vi "UIStep Execte UI Validate Input.vi"(10 "UI Setting":T1={"Embedded"=FALSE, "Size"=enum."Small", "Title"="", "Content"="", "Text Style"={"Font"="", "Size"=0.0, "Justification"=1, "TextColor"=0, "BGColor"=0, "Bold"=FALSE}, "Buttons"={"Button1"={"Label"="", "Size"=0.0, "TextColor"=0, "BGColor"=0, "Bold"=FALSE}, "Button2"={"Label"="", "Size"=0.0, "TextColor"=0, "BGColor"=0, "Bold"=FALSE}}, "Image"=path "", "Enable Input"=FALSE, "Input Validation"=""} {"Text Style"."Justification" items=["Left", "Center", "Right"]}, 11 "UI Control":T2) -> (2 "Valid out":bool, 3 "UI Control out":T2)   [LabVIEW 2015, in "UIStep.lvclass"]
uses:
  UIStep.lvclass
  <vilib>/regexp/Match Regular Expression.xnode
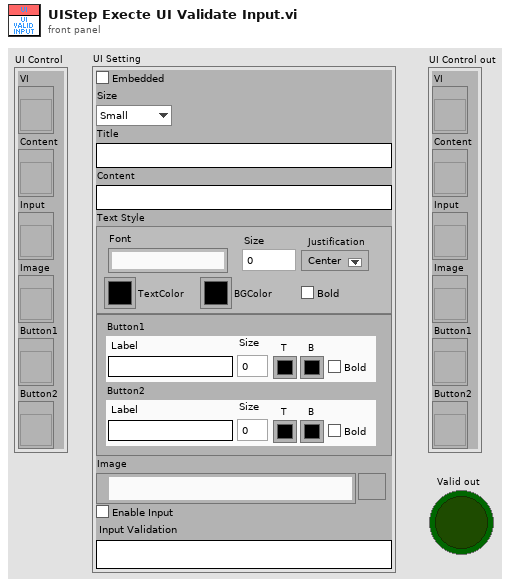
[diagram p1: front panel]
types:
  T1 = cluster{"Embedded":bool, "Size":enum16{"Small", "Middle", "Big"}, "Title":string, "Content":string, "Text Style":cluster{"Font":string, "Size":dbl, "Justification":u16, "TextColor":u32, "BGColor":u32, "Bold":bool}, "Buttons":cluster{"Button1":cluster{"Label":string, "Size":dbl, "TextColor":u32, "BGColor":u32, "Bold":bool}, "Button2":cluster{"Label":string, "Size":dbl, "TextColor":u32, "BGColor":u32, "Bold":bool}}, "Image":path, "Enable Input":bool, "Input Validation":string}
  T2 = cluster{"VI":refnum<vi>, "Content":refnum<vi>, "Input":refnum<vi>, "Image":refnum<vi>, "Button1":refnum<vi>, "Button2":refnum<vi>}
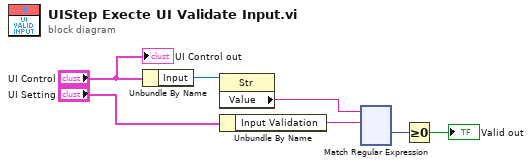
[diagram p0: block diagram]
diagram:
  n1 = Unbundle By Name("UI Control") -> ("Input"=w6:refnum<vi>)
  n2 = property class="Str"(reference=w6) -> ("Value"=w4:string)  [unwired: 1 in, 2 out]
  n3 = Unbundle By Name("UI Setting") -> ("Input Validation"=w3:string)
  n4 = xnode "Match Regular Expression"("input string"=w4, "regular expression"=w3) -> ("offset past match"=w2:i32)  [unwired: 4 in, 4 out]
  n5 = Greater Or Equal To 0?(x=w2) -> (x >= 0?=→"Valid out":bool)
  "UI Control out" <- "UI Control"
